vi "BatchRun.vi"() -> ()   [LabVIEW 2010]
panel:
  in  "stop":bool=TRUE
  out "waiting file list":string[](array[string])
  out "Running file":string
  in  "BatchFolder":path
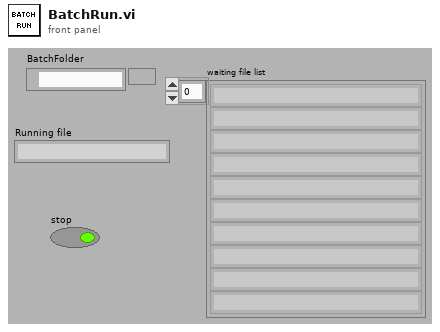
[diagram p1: front panel]
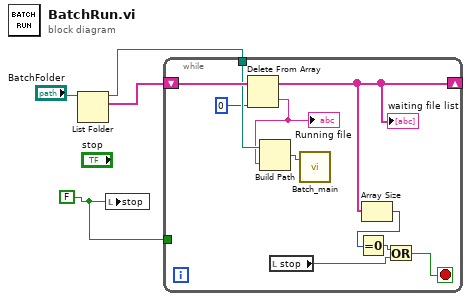
[diagram p0: block diagram]
diagram:
  w2 = FALSE
  n1 = List Folder(path="BatchFolder") -> (path out=w3:path, filenames=w1:string[])  [unwired: 3 in, 2 out]
  n2 = local write "stop"(w2) -> ()
  n3 = while {
    shift-right: [w11] -> _
    shift-left: w1 -> [w14]
    tunnel: w3 -> [w13]
    tunnel: w2 -> [_]
    stop <- w7 stop-if-true
    n4 = Delete From Array(array=w14, index=0) -> (deleted portion=w12:string, array with subset deleted=w11:string[])  [unwired: 1 in]
    "Running file" <- w12
    "waiting file list" <- w11
    n5 = Build Path(base path=w13, name or relative path=w12) -> (appended path=w5:path)
    n6 = local read "stop"() -> (w8:bool)
    n7 = call "Batch_main.vi"("ExpFilePath"=w5) -> ()  [unwired: 2 in]
    n8 = Array Size(array=w11) -> (size(s)=w10:i32)
    n9 = Equal To 0?(x=w10) -> (x = 0?=w9:bool)
    n10 = Or(x=w9, y=w8) -> (x .or. y?=w7:bool)
  }
